vi "String to Matlab String.vi"(8 "error in (no error)":errorcluster, 10 "Value":string, 11 "Variable name":string) -> (0 "error out":errorcluster, 3 "String":string)   [LabVIEW 2014, in "Matlab API.lvlib"]
uses:
  Matlab API.lvlib
panel:
  out "Array":u8[](array[numeric]) format="%x"
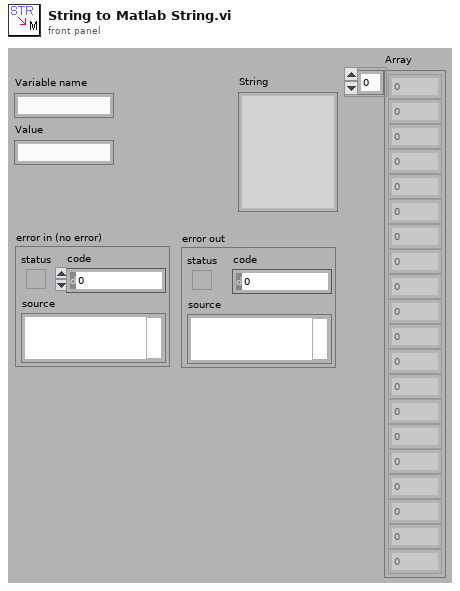
[diagram p1: front panel]
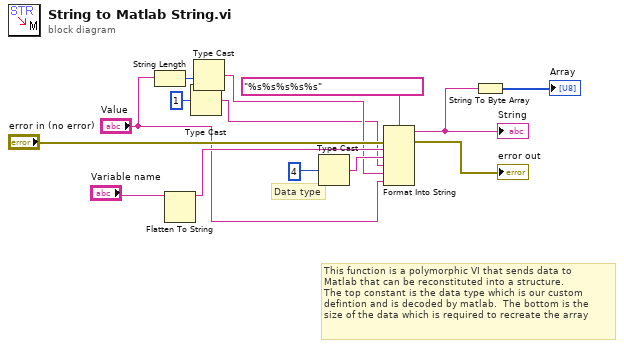
[diagram p0: block diagram]
diagram:
  # "Data type"
  # "This function is a polymorphic VI that sends data to\nMatlab that can be reconstituted into a structure.\nThe top constant is the data type which is our custom\ndefintion and is decoded by matlab.  The bottom is the\nsize of the data which is required to recreate the array"
  n1 = String Length(string="Value") -> (length=w3:i32)
  n2 = Flatten To String(anything="Variable name") -> (data string=w7:string)  [unwired: 1 in, 4 out]
  n3 = Type Cast(x=1) -> (*(type *) &x=w1:string)  [unwired: 1 out]
  n4 = Type Cast(x=w3) -> (*(type *) &x=w2:string)  [unwired: 1 out]
  n5 = Type Cast(x=4 ("input 2")) -> (*(type *) &x=w11:string)  [unwired: 1 out]
  n6 = Format Into String(format string="%s%s%s%s%s", error in="error in (no error)", w7, w11, w1, w2, "Value") -> (resulting string=w9:string, error out=→"error out":errorcluster)  [unwired: 1 in]
  "String" <- w9
  n7 = String To Byte Array(string=w9) -> (unsigned byte array=→"Array":u8[])
